vi "AO one shot.vi"() -> ()   [LabVIEW 2009, in "MicroDAQ.lvlib"]
uses:
  <instrlib>/MicroDAQ/MicroDAQ.lvlib
  <instrlib>/MicroDAQ/Tools/Analo Range Enum.ctl
  <instrlib>/MicroDAQ/Tools/Analog Channel Enum.ctl
  <instrlib>/MicroDAQ/Channel/Analog Output/Write NChan 1Sample 1D SGL.vi
  <instrlib>/MicroDAQ/Channel/Analog Output/Analog output.lvclass
panel:
  out "error out":errorcluster
  in  "Phisical channels":T1[](array[typedef])
  in  "Ranges":T2[](array[typedef])
  in  "data":sgl[](array[numeric])
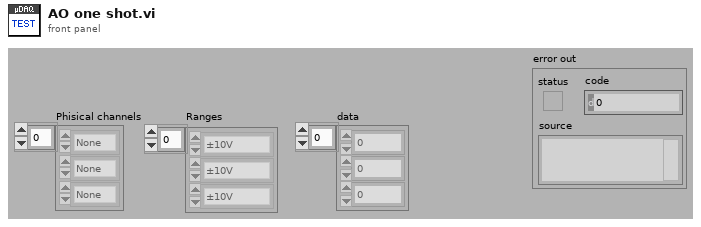
[diagram p1: front panel]
types:
  T1 = typedef "MicroDAQ.lvlib/Analog Channel Enum.ctl" = enum16{"None", "AO1", "AO2", "AO3", "AO4", "AO5", "AO6", "AO7", "AO8", "AO9", "AO10", "AO11", "AO12", "AO13", "AO14", "AO15", "AO16"}
  T2 = typedef "MicroDAQ.lvlib/Analo Range Enum.ctl" = enum16{"±10V", "0-10V", "±5V", "0-5V", "±5.12V", "±2.56V", "±2.5V", "±2V", "±1.24V", "±0.64V"}
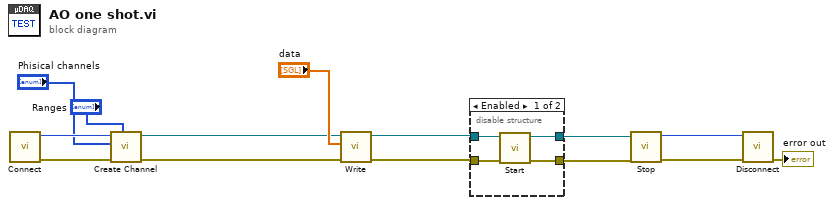
[diagram p0: block diagram]
diagram:
  n1 = call <instrlib>:"Connect.vi"() -> ("error out"=w12:errorcluster, "connection ID"=w13:i32)  [unwired: 10 in]
  n2 = call-poly <instrlib>:"Create Channel.vi"("Ranges"="Ranges", "error in (no error)"=w12, "Phisical channels"="Phisical channels", "Connection ID"=w13) -> ("error out"=w3:errorcluster, "Task Out"=w5:refnum<class "Analog output.lvclass">)  [unwired: 6 in]
  n3 = call-poly <instrlib>:"Write.vi"("error in (no error)"=w3, "data"="data", "Analog Output in"=w5) -> ("Analog Output out"=w4:refnum<class "Analog output.lvclass">)  [unwired: 7 in, 1 out]
  n4 = disable-structure shown="Enabled" {
    disable-tunnel: w4 -> [w15 w19]
    disable-tunnel: [w17 w19] -> w1
    disable-tunnel: w3 -> [w14 w18]
    disable-tunnel: [w16 w18] -> w2
    frame #0 {
      n5 = call-dynamic "Start.vi"("error in (no error)"=w14, "Analog Output in"=w15) -> ("error out"=w16:errorcluster, "Analog Output out"=w17:refnum<class "Analog output.lvclass">)  [unwired: 8 in]
    }
    frame #1 {
    }
  }
  n6 = call-dynamic "Stop.vi"("error in (no error)"=w2, "Analog Output in"=w1) -> ("error out"=w11:errorcluster, "connection ID"=w10:i32)  [unwired: 8 in]
  n7 = call <instrlib>:"Disconnect.vi"("error in (no error)"=w11, "connection ID"=w10) -> ("error out"=→"error out":errorcluster)  [unwired: 9 in]
